vi "VI Tree.vi"   [LabVIEW 2022 SP3, in "Agilent N934X Series.lvlib"]
doc: "This is the instrument driver for the Keysight (Agilent) N9342/43/44/22C. The VI Tree displays all the user-callable VIs of the instrument driver in an organized table."
uses:
  <instrlib>/Agilent N934X Series/Agilent N934X Series.lvlib
  <instrlib>/Agilent N934X Series/Public/Configure/Measurement/Configure Measurement (Adjacent Channel Power Ratio).vi
  <instrlib>/Agilent N934X Series/Public/Configure/Measurement/Configure Offset and Limits (Adjacent Channel Power).vi
  <instrlib>/Agilent N934X Series/Public/Configure/Configure Trace (Power Meter).vi
  <instrlib>/Agilent N934X Series/Public/Configure/Configure Frequency (Center Span).vi
  <instrlib>/Agilent N934X Series/Public/Data/Low Level/Fetch Measurement (Channel Power).vi
  <instrlib>/Agilent N934X Series/Public/Data/Read Measurement (Channel Power).vi
panel:
  # "(c) 2012 - 2025 National Instruments.  ALL RIGHTS RESERVED."
  # "SEE DIAGRAM\nFOR VI TREE."
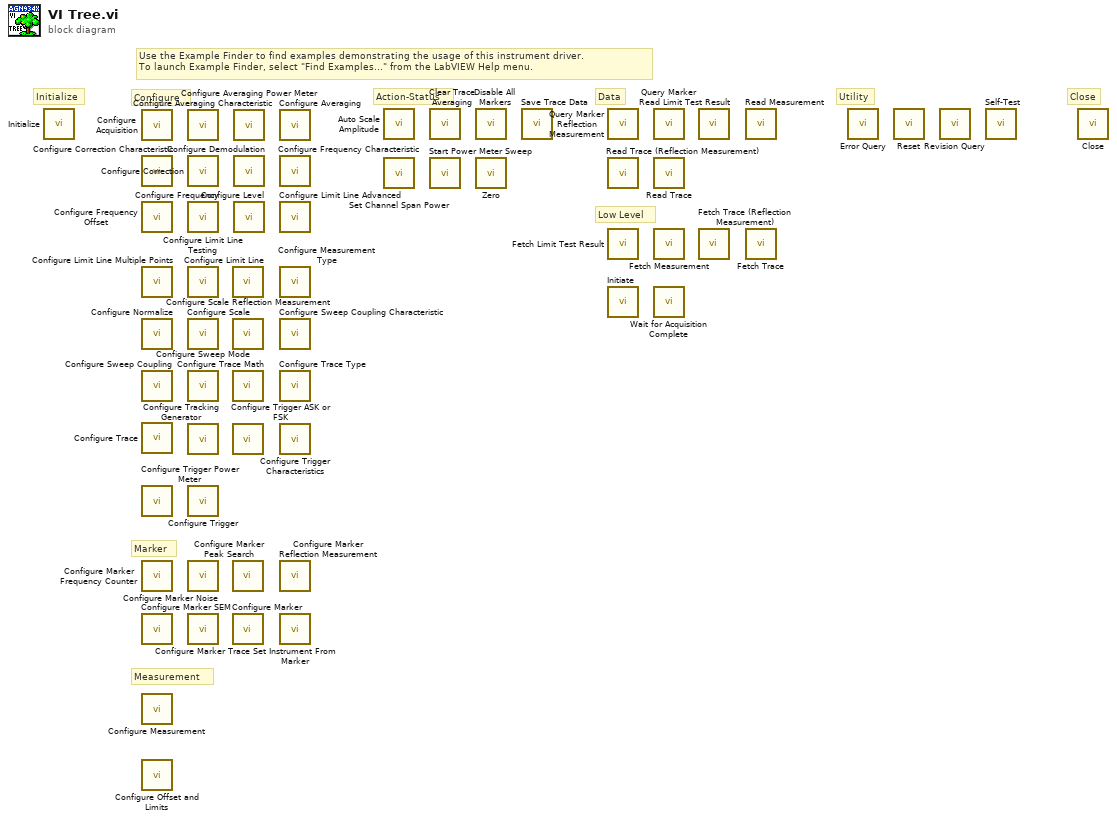
[diagram p0: block diagram]
diagram:
  # "Close"
  # "Utility"
  # "Low Level"
  # "Data"
  # "Measurement"
  # "Marker"
  # "Configure"
  # "Action-Status"
  # "Initialize"
  # "Use the Example Finder to find examples demonstrating the usage of this instrument driver.\nTo launch Example Finder, select \"Find Examples...\" from the LabVIEW Help menu."
  n1 = call <instrlib>:"Initialize.vi"() -> ()  [unwired: 10 in, 2 out]
  n2 = call <instrlib>:"Configure Acquisition.vi"() -> ()  [unwired: 14 in, 2 out]
  n3 = call <instrlib>:"Configure Correction Characteristic.vi"() -> ()  [unwired: 10 in, 2 out]
  n4 = call <instrlib>:"Configure Frequency Offset.vi"() -> ()  [unwired: 10 in, 2 out]
  n5 = call <instrlib>:"Configure Limit Line Multiple Points.vi"() -> ()  [unwired: 10 in, 2 out]
  n6 = call <instrlib>:"Configure Normalize.vi"() -> ()  [unwired: 10 in, 2 out]
  n7 = call <instrlib>:"Configure Sweep Coupling.vi"() -> ()  [unwired: 14 in, 2 out]
  n8 = call-poly <instrlib>:"Configure Trace.vi"() -> ()  [unwired: 10 in, 2 out]
  n9 = call <instrlib>:"Configure Trigger Power Meter.vi"() -> ()  [unwired: 14 in, 2 out]
  n10 = call <instrlib>:"Configure Marker Frequency Counter.vi"() -> ()  [unwired: 10 in, 2 out]
  n11 = call <instrlib>:"Configure Marker SEM.vi"() -> ()  [unwired: 10 in, 2 out]
  n12 = call-poly <instrlib>:"Configure Measurement.vi"() -> ()  [unwired: 14 in, 2 out]
  n13 = call-poly <instrlib>:"Configure Offset and Limits.vi"() -> ()  [unwired: 14 in, 2 out]
  n14 = call <instrlib>:"Configure Averaging Characteristic.vi"() -> ()  [unwired: 10 in, 2 out]
  n15 = call <instrlib>:"Configure Correction.vi"() -> ()  [unwired: 10 in, 2 out]
  n16 = call-poly <instrlib>:"Configure Frequency.vi"() -> ()  [unwired: 14 in, 2 out]
  n17 = call <instrlib>:"Configure Limit Line Testing.vi"() -> ()  [unwired: 14 in, 2 out]
  n18 = call <instrlib>:"Configure Scale.vi"() -> ()  [unwired: 14 in, 2 out]
  n19 = call <instrlib>:"Configure Sweep Mode.vi"() -> ()  [unwired: 10 in, 2 out]
  n20 = call <instrlib>:"Configure Tracking Generator.vi"() -> ()  [unwired: 10 in, 2 out]
  n21 = call <instrlib>:"Configure Trigger.vi"() -> ()  [unwired: 10 in, 2 out]
  n22 = call <instrlib>:"Configure Marker Noise.vi"() -> ()  [unwired: 10 in, 2 out]
  n23 = call <instrlib>:"Configure Marker Trace.vi"() -> ()  [unwired: 10 in, 2 out]
  n24 = call <instrlib>:"Configure Limit Line.vi"() -> ()  [unwired: 10 in, 2 out]
  n25 = call <instrlib>:"Configure Scale Reflection Measurement.vi"() -> ()  [unwired: 10 in, 2 out]
  n26 = call <instrlib>:"Configure Trace Math.vi"() -> ()  [unwired: 14 in, 2 out]
  n27 = call <instrlib>:"Configure Trigger ASK or FSK.vi"() -> ()  [unwired: 10 in, 2 out]
  n28 = call <instrlib>:"Configure Marker Peak Search.vi"() -> ()  [unwired: 14 in, 2 out]
  n29 = call <instrlib>:"Configure Marker.vi"() -> ()  [unwired: 14 in, 2 out]
  n30 = call <instrlib>:"Configure Averaging Power Meter.vi"() -> ()  [unwired: 10 in, 2 out]
  n31 = call <instrlib>:"Configure Demodulation.vi"() -> ()  [unwired: 10 in, 2 out]
  n32 = call <instrlib>:"Configure Level.vi"() -> ()  [unwired: 14 in, 2 out]
  n33 = call <instrlib>:"Configure Averaging.vi"() -> ()  [unwired: 14 in, 2 out]
  n34 = call <instrlib>:"Configure Frequency Characteristic.vi"() -> ()  [unwired: 10 in, 2 out]
  n35 = call <instrlib>:"Configure Limit Line Advanced.vi"() -> ()  [unwired: 10 in, 2 out]
  n36 = call <instrlib>:"Configure Measurement Type.vi"() -> ()  [unwired: 10 in, 2 out]
  n37 = call <instrlib>:"Configure Sweep Coupling Characteristic.vi"() -> ()  [unwired: 14 in, 2 out]
  n38 = call <instrlib>:"Configure Trace Type.vi"() -> ()  [unwired: 10 in, 2 out]
  n39 = call <instrlib>:"Configure Trigger Characteristics.vi"() -> ()  [unwired: 10 in, 2 out]
  n40 = call <instrlib>:"Configure Marker Reflection Measurement.vi"() -> ()  [unwired: 10 in, 2 out]
  n41 = call <instrlib>:"Set Instrument From Marker.vi"() -> ()  [unwired: 10 in, 2 out]
  n42 = call <instrlib>:"Auto Scale Amplitude.vi"() -> ()  [unwired: 10 in, 2 out]
  n43 = call <instrlib>:"Set Channel Span Power.vi"() -> ()  [unwired: 10 in, 2 out]
  n44 = call <instrlib>:"Clear Trace Averaging.vi"() -> ()  [unwired: 10 in, 2 out]
  n45 = call <instrlib>:"Start Power Meter Sweep.vi"() -> ()  [unwired: 10 in, 2 out]
  n46 = call <instrlib>:"Disable All Markers.vi"() -> ()  [unwired: 10 in, 2 out]
  n47 = call <instrlib>:"Zero.vi"() -> ()  [unwired: 10 in, 2 out]
  n48 = call <instrlib>:"Save Trace Data.vi"() -> ()  [unwired: 10 in, 2 out]
  n49 = call <instrlib>:"Query Marker Reflection Measurement.vi"() -> ()  [unwired: 8 in, 4 out]
  n50 = call <instrlib>:"Read Trace (Reflection Measurement).vi"() -> ()  [unwired: 9 in, 3 out]
  n51 = call <instrlib>:"Fetch Limit Test Result.vi"() -> ()  [unwired: 9 in, 3 out]
  n52 = call <instrlib>:"Initiate.vi"() -> ()  [unwired: 10 in, 2 out]
  n53 = call <instrlib>:"Query Marker.vi"() -> ()  [unwired: 9 in, 3 out]
  n54 = call <instrlib>:"Read Trace.vi"() -> ()  [unwired: 9 in, 3 out]
  n55 = call-poly <instrlib>:"Fetch Measurement.vi"() -> ()  [unwired: 12 in, 4 out]
  n56 = call <instrlib>:"Wait for Acquisition Complete.vi"() -> ()  [unwired: 10 in, 2 out]
  n57 = call <instrlib>:"Read Limit Test Result.vi"() -> ()  [unwired: 9 in, 3 out]
  n58 = call <instrlib>:"Fetch Trace (Reflection Measurement).vi"() -> ()  [unwired: 9 in, 3 out]
  n59 = call-poly <instrlib>:"Read Measurement.vi"() -> ()  [unwired: 12 in, 4 out]
  n60 = call <instrlib>:"Fetch Trace.vi"() -> ()  [unwired: 9 in, 3 out]
  n61 = call <instrlib>:"Error Query.vi"() -> ()  [unwired: 8 in, 4 out]
  n62 = call <instrlib>:"Reset.vi"() -> ()  [unwired: 10 in, 2 out]
  n63 = call <instrlib>:"Revision Query.vi"() -> ()  [unwired: 8 in, 4 out]
  n64 = call <instrlib>:"Self-Test.vi"() -> ()  [unwired: 8 in, 4 out]
  n65 = call <instrlib>:"Close.vi"() -> ()  [unwired: 11 in, 1 out]
